vi "while.vi"(0 "error in":errorcluster, 2 "adress string":string) -> (1 "Phase Shift":dbl, 3 "error out":errorcluster, 4 "Errror U2":dbl, 5 "Error PS":dbl, 6 "Amplitude":dbl format="%#_10e", 7 "Error  Amp":dbl, 8 "U2":dbl, 9 "U1":dbl, 10 "Error U1":dbl)   [LabVIEW 2010]
uses:
  <vilib>/Analysis/NI_AALBase.lvlib
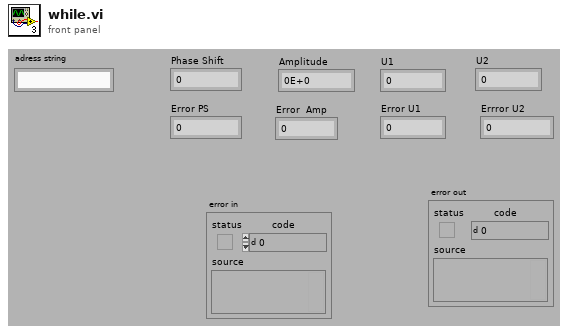
[diagram p1: front panel]
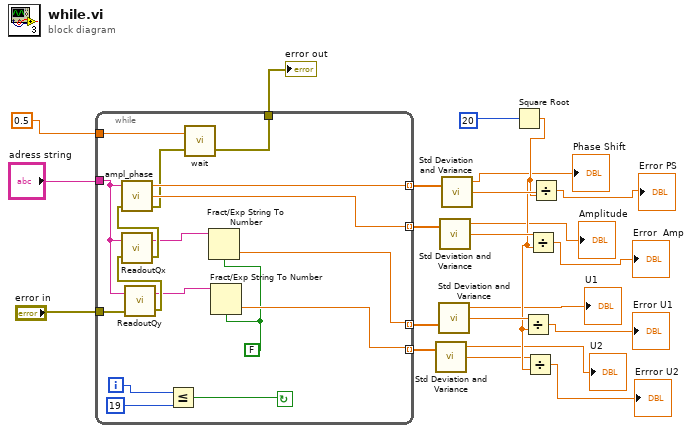
[diagram p0: block diagram]
diagram:
  n1 = while {
    tunnel: "adress string" -> [w32]
    tunnel: "error in" -> [w35]
    tunnel: [w38] -> w20 mode=indexing
    tunnel: [w37] -> w19 mode=indexing
    tunnel: [w29] -> w17 mode=indexing
    tunnel: [w28] -> w18 mode=indexing
    tunnel: 0.5 -> [w26]
    tunnel: [w25] -> w2
    i -> [w24]
    stop <- w36 continue-if-true
    w23 = FALSE
    n2 = call "ReadoutQy.vi"("error in"=w35, "address string"=w32) -> ("error out"=w34:errorcluster, "String"=w30:string)
    n3 = call "ReadoutQx.vi"("error in"=w34, "address string"=w32) -> ("error out"=w33:errorcluster, "String"=w31:string)
    n4 = call "ampl_phase.vi"("error in"=w33, "adress string"=w32) -> ("error out"=w27:errorcluster, "amplitude"=w37:dbl, "phase shi ft"=w38:dbl)  [unwired: 1 in]
    n5 = Less Or Equal?(x=w24, y=19) -> (x <= y?=w36:bool)
    n6 = call "wait.vi"("error in"=w27, "Wartezeit in Sek"=w26) -> ("error out"=w25:errorcluster)  [unwired: 1 in]
    n7 = Fract/Exp String To Number(use system decimal point (T)=w23, string=w31) -> (number=w28:dbl)  [unwired: 2 in, 1 out]
    n8 = Fract/Exp String To Number(use system decimal point (T)=w23, string=w30) -> (number=w29:dbl)  [unwired: 2 in, 1 out]
  }
  "error out" <- w2
  n9 = call <vilib>:"Std Deviation and Variance.vi"("X"=w17) -> ("mean"=→"U2":dbl, "standard deviation"=w11:dbl)  [unwired: 1 in, 1 out]
  n10 = call <vilib>:"Std Deviation and Variance.vi"("X"=w18) -> ("mean"=→"U1":dbl, "standard deviation"=w13:dbl)  [unwired: 1 in, 1 out]
  n11 = call <vilib>:"Std Deviation and Variance.vi"("X"=w19) -> ("mean"=→"Amplitude":dbl, "standard deviation"=w14:dbl)  [unwired: 1 in, 1 out]
  n12 = call <vilib>:"Std Deviation and Variance.vi"("X"=w20) -> ("mean"=→"Phase Shift":dbl, "standard deviation"=w16:dbl)  [unwired: 1 in, 1 out]
  n13 = Square Root(x=20) -> (sqrt(x)=w12:dbl)
  n14 = Divide(x=w13, y=w12) -> (x/y=→"Error U1":dbl)
  n15 = Divide(x=w11, y=w12) -> (x/y=→"Errror U2":dbl)
  n16 = Divide(x=w14, y=w12) -> (x/y=→"Error  Amp":dbl)
  n17 = Divide(x=w16, y=w12) -> (x/y=→"Error PS":dbl)
